vi "Initialize-object.vi"(7 "Main VI ref":refnum<vi>, 8 "error in (no error)":errorcluster, 9 "Client channel":refnum<queue>, 10 "Server channel":refnum<queue>) -> (0 "error out":errorcluster, 3 "Object ref out":T1)   [LabVIEW 2013, in "PowderDeposition.lvlib" / "PD-Main.lvclass"]
uses:
  PD-Main.lvclass
  Object-reference.ctl
  SA-SLMAPI/Sources/Message.lvclass
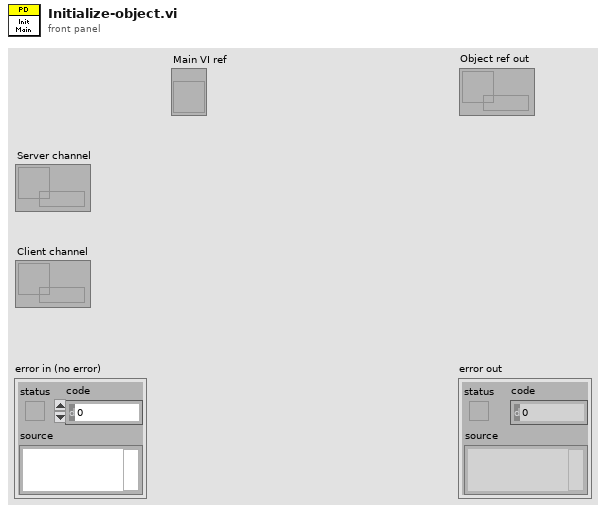
[diagram p1: front panel]
types:
  T1 = typedef "PowderDeposition.lvlib/PD-Main.lvclass/Object-reference.ctl" = refnum<data-value>
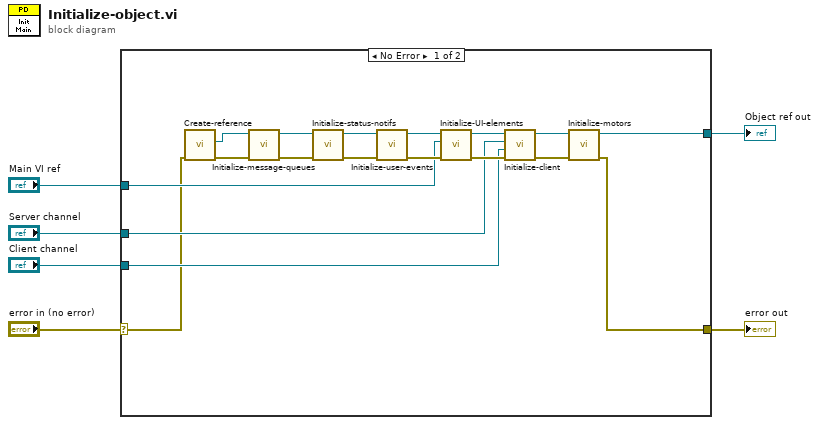
[diagram p0: block diagram]
diagram:
  n1 = case shown="No Error" "error in (no error)" {
    selector: "error in (no error)" -> [w7 w25]
    tunnel: [w13 w25] -> w5
    tunnel: [w10 _] -> w4
    tunnel: "Main VI ref" -> [w16 _]
    tunnel: "Server channel" -> [w15 _]
    tunnel: "Client channel" -> [w14 _]
    frame No Error {
      n2 = call "Create-reference.vi"("error in (no error)"=w7) -> ("error out"=w8:errorcluster, "Data ref"=w9:T1)  [unwired: 8 in, 1 out]
      n3 = call "Initialize-message-queues.vi"("error in (no error)"=w8, "Object ref in"=w9) -> ("error out"=w20:errorcluster, "Object ref out"=w24:T1)  [unwired: 8 in]
      n4 = call "Initialize-status-notifs.vi"("error in (no error)"=w20, "Object ref in"=w24) -> ("error out"=w19:errorcluster, "Object ref out"=w23:T1)  [unwired: 8 in]
      n5 = call "Initialize-user-events.vi"("error in (no error)"=w19, "Object ref in"=w23) -> ("error out"=w18:errorcluster, "Object ref out"=w22:T1)  [unwired: 8 in]
      n6 = call "Initialize-UI-elements.vi"("error in (no error)"=w18, "Main VI ref"=w16, "Object ref in"=w22) -> ("error out"=w17:errorcluster, "Object ref out"=w21:T1)  [unwired: 7 in]
      n7 = call "Initialize-client.vi"("error in (no error)"=w17, "Client channel"=w14, "Server channel"=w15, "Object ref in"=w21) -> ("error out"=w12:errorcluster, "Object ref out"=w11:T1)  [unwired: 6 in]
      n8 = call "Initialize-motors.vi"("error in (no error)"=w12, "Object ref in"=w11) -> ("error out"=w13:errorcluster, "Object ref out"=w10:T1)  [unwired: 8 in]
    }
    frame Error {
    }
  }
  "error out" <- w5
  "Object ref out" <- w4
